vi "Helper Loop.vi"(8 "error in (no error)":errorcluster, 11 "RFSA DAQ in":refnum<class "RFSA DAQ.lvclass">) -> ()   [LabVIEW 2025, in "RFSA DAQ.lvlib" / "RFSA DAQ.lvclass"]
uses:
  RFSA DAQ.lvclass
  Helper Loop State.ctl
  <vilib>/Natan Biesmans/G2CPU GPU and CPU HPC Toolkit/G2CPU Libraries/Async IO/DMA Manager/DMA Manager.lvclass
  Configure VST.ctl
  <vilib>/Platform/TimedLoop/XDataNode/timing_clust.ctl
  <vilib>/Platform/TimedLoop/XDataNode/nitl_modes.ctl
  <vilib>/Platform/TimedLoop/XDataNode/wakeup.ctl
  RFSA DAQ.lvclass/RFSA DAQ.ctl
  <instrlib>/niRFSA/niRFSA.llb/niRFSA Acquisition Types.ctl
  Helper Loop Message.ctl
  Helper Loop Type.ctl
  TDMS DAQ/TDMS DAQ/Filled Buffers.ctl
  <vilib>/ActorFramework/Actor/Actor.lvclass/Actor.ctl
  <vilib>/ActorFramework/Message Enqueuer/Message Enqueuer.lvclass/Message Enqueuer.ctl
  DAQ Interface/DAQ Interface Messages/Process Filled Buffer Msg/Process Filled Buffer Msg.lvclass/Process Filled Buffer Msg.ctl
  780f3a39-6c74-4c42-b9e6-83f74691e199.vi
  780f3a39-6c74-4c42-b9e6-83f74691e199.vi/8445960e-929f-4715-bef2-3345fde3aa58.vi
  780f3a39-6c74-4c42-b9e6-83f74691e199.vi/206fbf6d-c74b-456c-96d5-ad8d28d1ffd8.vi
  780f3a39-6c74-4c42-b9e6-83f74691e199.vi/4cbfaf14-3946-45e6-aec4-337dfce7590f.vi
  780f3a39-6c74-4c42-b9e6-83f74691e199.vi/3076a2b9-925c-4d87-a949-889053232e05.vi
  <vilib>/ActorFramework/Message Enqueuer/Init from Existing Queue.vi
  <vilib>/ActorFramework/Message Enqueuer/Enqueue.vi
  <vilib>/Natan Biesmans/G2CPU GPU and CPU HPC Toolkit/G2CPU Libraries/Arrays/1DArray/s16/1D Array s16.lvclass
  DAQ Interface/DAQ Interface Messages/Process Filled Buffer Msg/Process Filled Buffer Msg.lvclass
  <instrlib>/niRFSA/niRFSA.llb/niRFSA Fetch IQ (1D I16 Data Ref).vi
  <vilib>/Natan Biesmans/G2CPU GPU and CPU HPC Toolkit/G2CPU Libraries/Runtime Licensing/G2CPU License Check.vi
  <vilib>/Natan Biesmans/G2CPU GPU and CPU HPC Toolkit/G2CPU Libraries/Manage Environment/G2CPU Get Backend.vi
  <vilib>/Utility/error.llb/Error Cluster From Error Code.vi
  <vilib>/Natan Biesmans/G2CPU GPU and CPU HPC Toolkit/G2CPU Libraries/Manage Environment/Find AF DLL.vi
  <vilib>/Natan Biesmans/G2CPU GPU and CPU HPC Toolkit/ArrayFire Driver/VIs/Run as Multi Device.vi
  <vilib>/Natan Biesmans/G2CPU GPU and CPU HPC Toolkit/G2CPU Libraries/Arrays/Array/G2CPU Set Array Pointer.vi
  <resource>/Natan Biesmans/G2CPU GPU and CPU HPC Toolkit/Garbage Collector/G2CPU DMAGarbageCollectorFGV.vi
  <vilib>/ActorFramework/Message Priority Queue/Priority Enqueue.vi
  <vilib>/platform/TimedLoop/XDataNode/XDataNode.xnode
  <vilib>/Natan Biesmans/G2CPU GPU and CPU HPC Toolkit/G2CPU Libraries/Arrays/Array/Array Prototype.lvclass
  <vilib>/ActorFramework/Message Enqueuer/Message Enqueuer.lvclass
  <vilib>/Platform/TimedLoop/XDataNode/XDNodeRunTimeDep.lvlib
  DAQ Interface/DAQ Interface/DAQ Interface.lvclass
  <vilib>/ActorFramework/Actor/Actor.lvclass
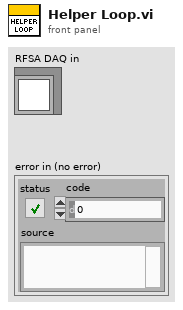
[diagram p1: front panel]
types:
  T1 = typedef "RFSA DAQ.lvlib/RFSA DAQ.lvclass/Helper Loop State.ctl" = cluster{"VST Config":T2, "DMA Manager":refnum<class "DMA Manager.lvclass">, "VST Handle":refnum<k15>, "Stop":bool}
  T2 = typedef "RFSA DAQ.lvlib/RFSA DAQ.lvclass/Configure VST.ctl" = cluster{"Samples to Read per Block":i32, "IQ rate (S/s)":dbl, "Carrier Frequency (Hz)":dbl, "Reference Level (dBm)":dbl, "Resource Name":refnum<k15>, "Clock Source":refnum<k15>, "Host DMA Buffer Size":i64}
  T3 = typedef "RFSA DAQ.lvlib/RFSA DAQ.lvclass/Helper Loop Message.ctl" = cluster{"Type":T4, "Payload":variant}
  T4 = typedef "RFSA DAQ.lvlib/RFSA DAQ.lvclass/Helper Loop Type.ctl" = enum16{"Configure", "Start", "Do", "Stop", "Clean", "Close"}
  T5 = typedef "DAQ Interface.lvlib/DAQ Interface.lvclass/Filled Buffers.ctl" = cluster{"DMA Manager":refnum<class "DMA Manager.lvclass">, "DMA Memory":refnum<data-value>, "Gain":dbl, "dt":dbl, "f0":dbl}
  T6 = typedef "XDNodeRunTimeDep.lvlib/timing_clust.ctl" = cluster{"Expected End [f-1]":u64, "Actual End [f-1]":u64, "Finished Late? [f-1]":bool, "Expected End [i-1]":u64, "Actual End [i-1]":u64, "Finished Late? [i-1]":bool, "Expected Start [i]":u64, "Actual Start [i]":u64, "Expected Start [f]":u64, "Actual Start [f]":u64, "Source Name":string, "Structure Name":string, "Period":i64, "Deadline":i64, "Offset":i64, "Start":i64, "Priority":i32, "Timeout":i32, "Mode":T7, "Wakeup Reason":T8, "Error":errorcluster, "Source Type":string, "Secondary Source Type":string, "Global End Time":u64, "Global Start Time":u64, "Frame Duration":u64, "Iteration Duration":u64, "Assigned CPU":i32, "I/O Scan Engine Mode":u32}
  T7 = typedef "XDNodeRunTimeDep.lvlib/nitl_modes.ctl" = enum32{"No Change", "Process missed periods, maintain original phase", "Discard missed periods, maintain original phase", "Process missed periods, ignore original phase", "Discard missed periods, ignore original phase"}
  T8 = typedef "XDNodeRunTimeDep.lvlib/wakeup.ctl" = enum32{"Normal", "Aborted", "Asynchronous wakeup", "Timing source error", "Timed loop error", "Timeout"}
  T9 = typedef "niRFSA Acquisition Types.ctl" = i32
  T10 = typedef "niRFSA wfmInfo.ctl" = cluster{"absolute timestamp":dbl, "relative timestamp":dbl, "dt":dbl, "actual samples read":i64, "offset":dbl, "gain":dbl, "reserved1":dbl, "reserved2":dbl}
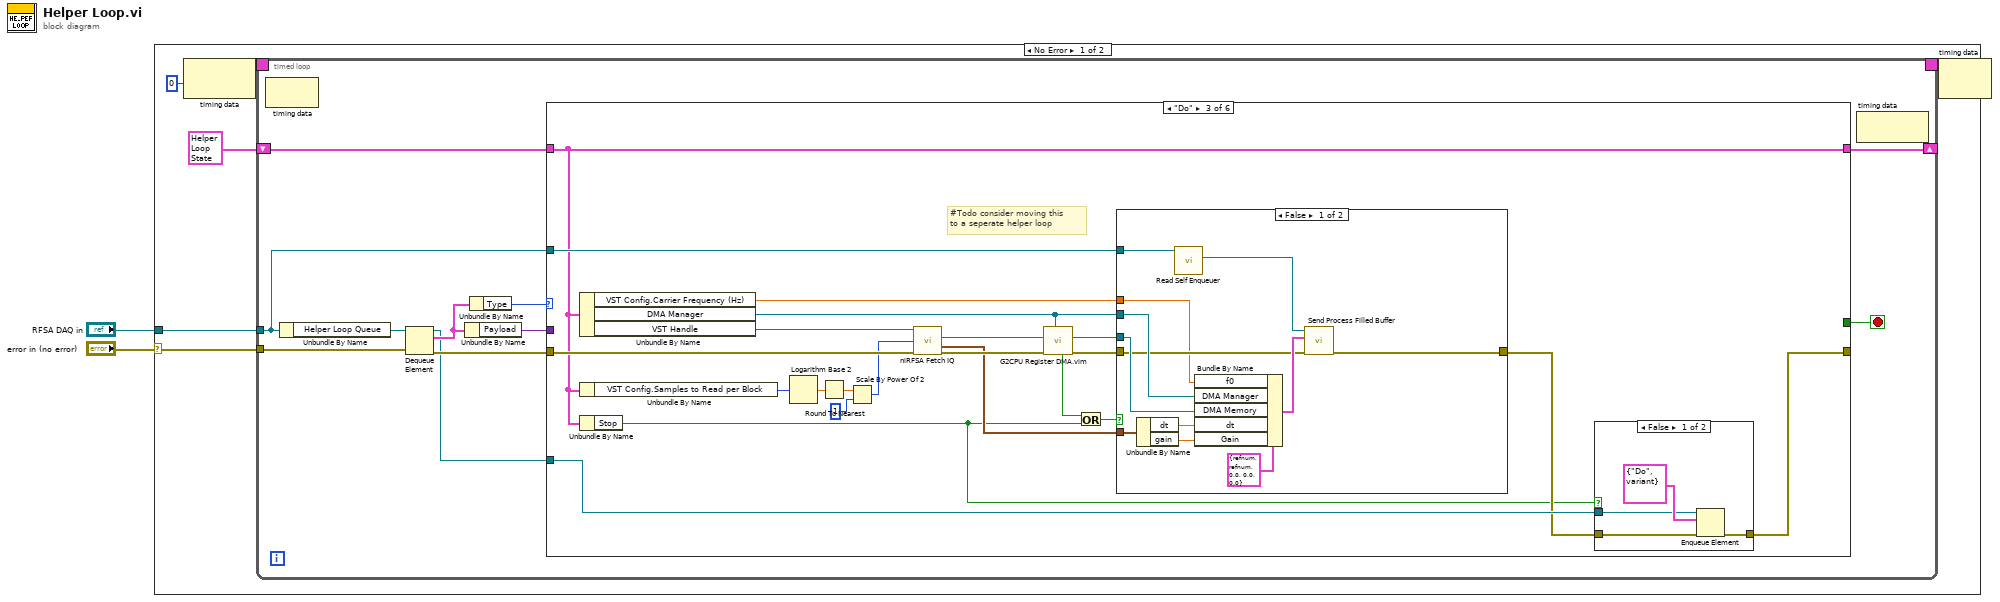
[diagram p0: block diagram]
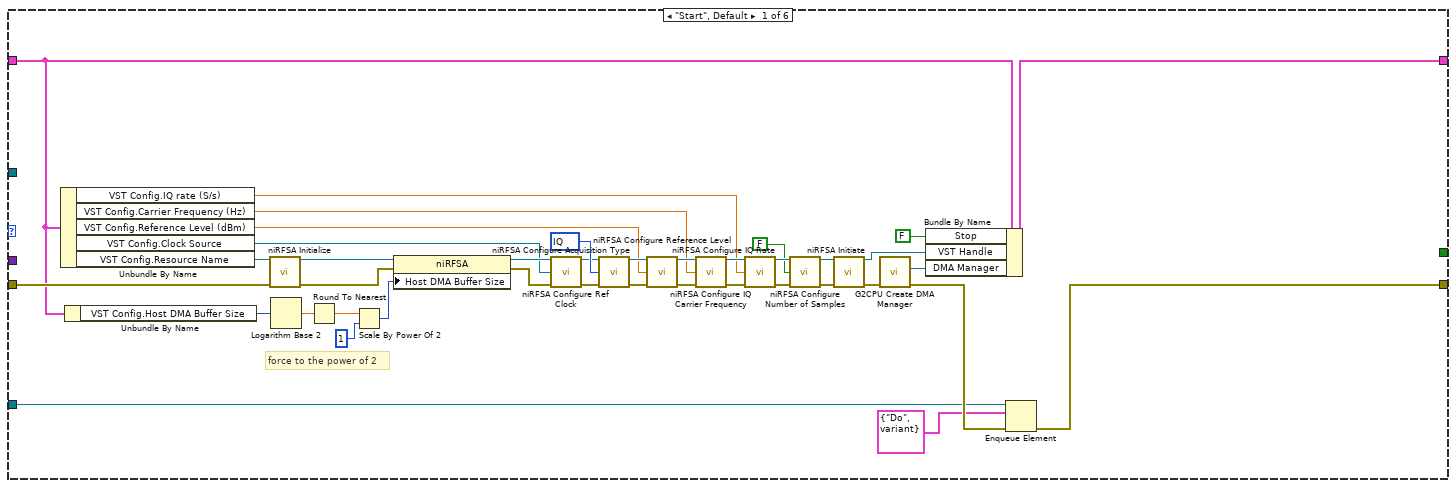
[diagram p2: hidden frame]
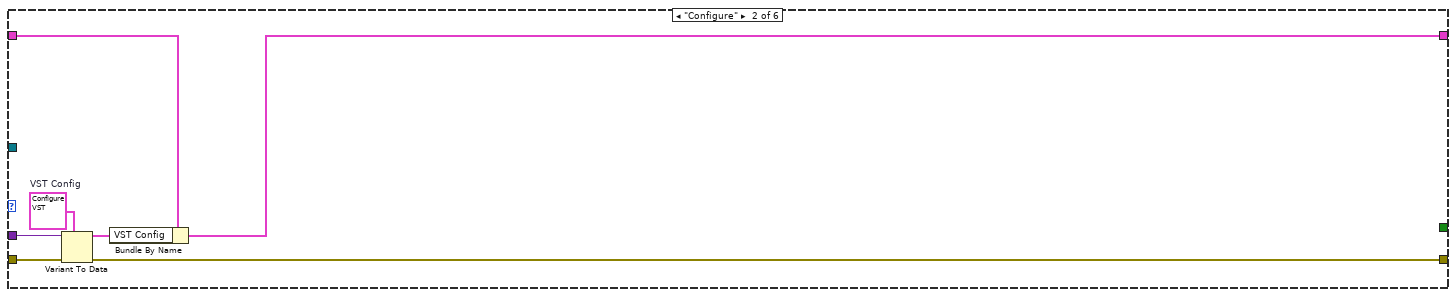
[diagram p3: hidden frame]
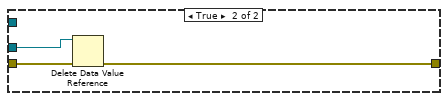
[diagram p5: hidden frame]
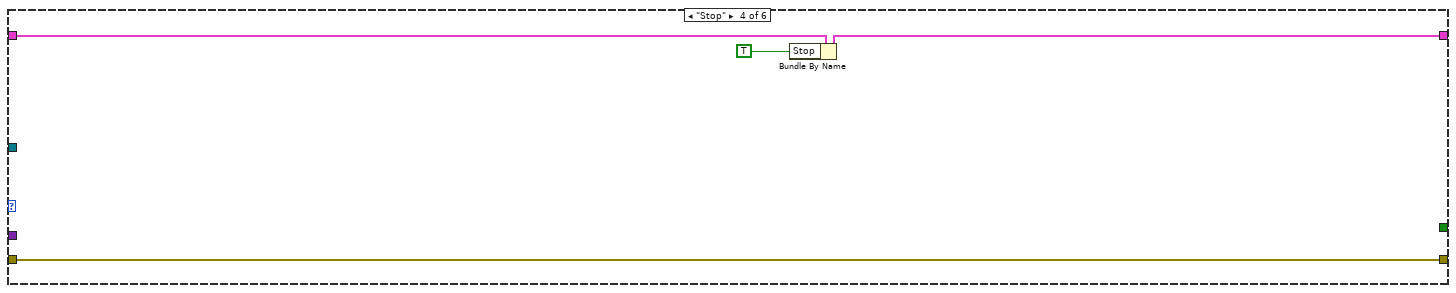
[diagram p6: hidden frame]
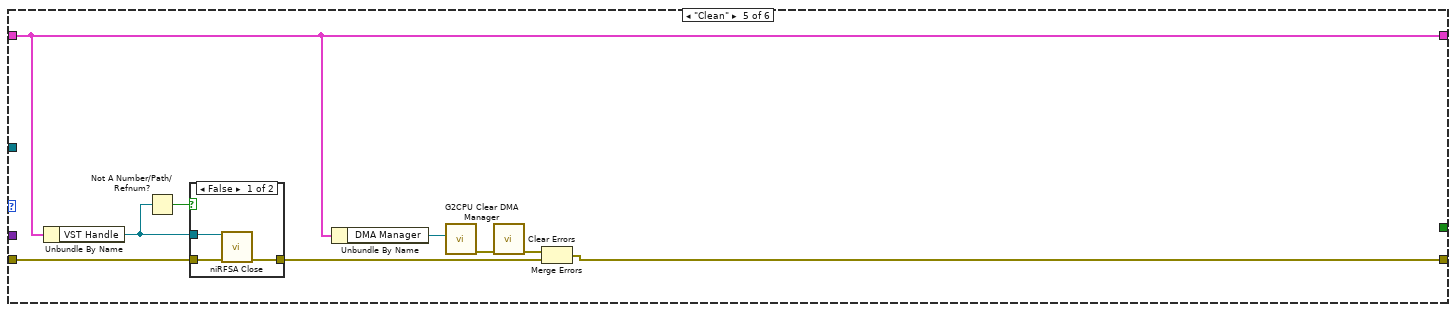
[diagram p7: hidden frame]
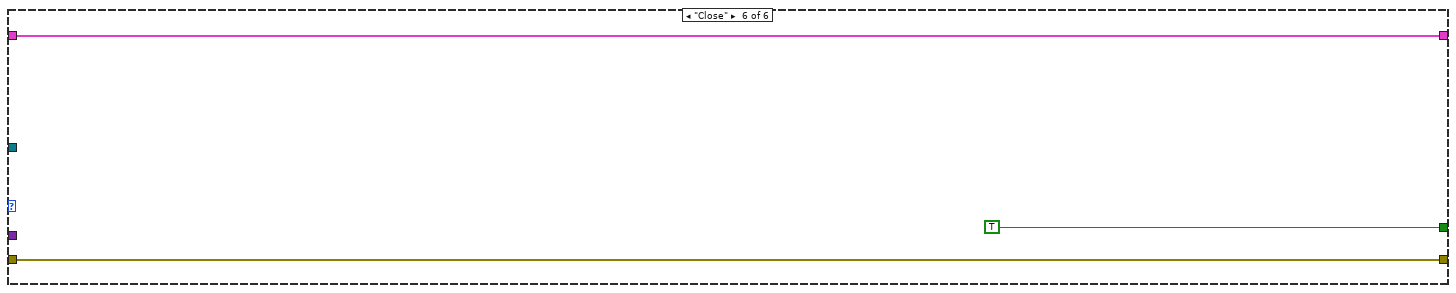
[diagram p9: hidden frame]
diagram:
  n1 = case shown="No Error" "error in (no error)" {
    selector: "error in (no error)" -> [w5 _]
    tunnel: "RFSA DAQ in" -> [w6 _]
    frame No Error {
      n2 = node-c288(i64 0 ("Period")) -> (w8:T6)
      n3 = timed-loop {
        timing: w8 -> [_]
        timing-out: [_] -> w7
        tunnel: w6 -> [w10]
        tunnel: w5 -> [w17]
        shift-right: [w12] -> _
        shift-left: T1 {"VST Config"={"Samples to Read per Block"=33554432, "IQ rate (S/s)"=1250000000.0, "Carrier Frequency (Hz)"=1000000000.0, "Reference Level (dBm)"=0.0, "Resource Name"="RFSA", "Clock Source"="OnboardClock", "Host DMA Buffer Size"=2000000000}, "DMA Manager"=refnum, "VST Handle"="", "Stop"=FALSE} ("State") -> [w11]
        stop <- w13 stop-if-true
        n4 = node-c288() -> ()  [unwired: 1 in, 1 out]
        n5 = Unbundle By Name(w10) -> ("Helper Loop Queue"=w19:refnum<queue>)
        n6 = Dequeue Element(queue=w19, error in (no error)=w17) -> (queue out=w9:refnum<queue>, element=w18:T3, error out=w15:errorcluster)  [unwired: 1 in, 1 out]
        n7 = Unbundle By Name(w18) -> ("Payload"=w14:variant)
        n8 = Unbundle By Name(w18) -> ("Type"=w16:T4)
        n9 = case shown="\"Do\"" w16 {
          tunnel: [w22 w62 w68 w110 w115 w127] -> _
          tunnel: w15 -> [w35 w63 w87 w110 w120 w127]
          tunnel: w14 -> [_ w64 _ _ _ _]
          tunnel: [_ _ _ _ _ TRUE] -> w13
          tunnel: [w27 w60 w71 w109 w116 w125] -> w12
          tunnel: w11 -> [w33 w61 w71 w111 w116 w125]
          tunnel: w10 -> [_ _ w74 _ _ _]
          tunnel: w9 -> [w21 _ w70 _ _ _]
          frame "Start", Default {
            w54 = T9 100 items=["IQ"=100, "Spectrum"=101] ("acquisition type")
            # "force to the power of 2"
            n10 = Unbundle By Name(w33) -> ("VST Config.IQ rate (S/s)"=w30:dbl, "VST Config.Carrier Frequency (Hz)"=w28:dbl, "VST Config.Reference Level (dBm)"=w29:dbl, "VST Config.Clock Source"=w31:refnum<k15>, "VST Config.Resource Name"=w34:refnum<k15>)
            n11 = Unbundle By Name(w33) -> ("VST Config.Host DMA Buffer Size"=w32:i64)
            n12 = call <instrlib>:"niRFSA Initialize.vi"("resource name"=w34, "error in"=w35) -> ("instrument handle out"=w45:refnum<k15>, "error out"=w38:errorcluster)  [unwired: 12 in]
            n13 = Logarithm Base 2(1:w32) -> (0:w39:dbl)
            n14 = Round To Nearest(number=w39) -> (nearest integer value=w40:dbl)
            n15 = Scale By Power Of 2(n=w40, x=u64 1) -> (x*2^n=w36:u64)
            n16 = property class="niRFSA"(reference=w45, error in=w38, "Host DMA Buffer Size"=w36) -> (reference out=w43:refnum<k15>, error out=w37:errorcluster)
            n17 = call <instrlib>:"niRFSA Configure Ref Clock.vi"("instrument handle"=w43, "clock source"=w31, "error in"=w37) -> ("instrument handle out"=w44:refnum<k15>, "error out"=w46:errorcluster)  [unwired: 11 in]
            n18 = call <instrlib>:"niRFSA Configure Acquisition Type.vi"("instrument handle"=w44, "acquisition type"=w54, "error in"=w46) -> ("instrument handle out"=w56:refnum<k15>, "error out"=w55:errorcluster)  [unwired: 11 in]
            n19 = call <instrlib>:"niRFSA Configure Reference Level.vi"("instrument handle"=w56, "reference level (dBm)"=w29, "error in"=w55) -> ("instrument handle out"=w57:refnum<k15>, "error out"=w58:errorcluster)  [unwired: 11 in]
            n20 = call <instrlib>:"niRFSA Configure IQ Carrier Frequency.vi"("instrument handle"=w57, "carrier frequency"=w28, "error in"=w58) -> ("instrument handle out"=w48:refnum<k15>, "error out"=w49:errorcluster)  [unwired: 11 in]
            n21 = call <instrlib>:"niRFSA Configure IQ Rate.vi"("instrument handle"=w48, "IQ rate (S/s)"=w30, "error in"=w49) -> ("instrument handle out"=w50:refnum<k15>, "error out"=w51:errorcluster)  [unwired: 11 in]
            n22 = call <instrlib>:"niRFSA Configure Number of Samples.vi"("instrument handle"=w50, "number of samples is finite"=FALSE, "error in"=w51) -> ("instrument handle out"=w53:refnum<k15>, "error out"=w52:errorcluster)  [unwired: 11 in]
            n23 = call <instrlib>:"niRFSA Initiate.vi"("instrument handle"=w53, "error in"=w52) -> ("instrument handle out"=w25:refnum<k15>, "error out"=w42:errorcluster)  [unwired: 12 in]
            n24 = call <vilib>:"G2CPU Create DMA Manager.vi"("error in (no error)"=w42) -> ("error out"=w23:errorcluster, "DMA Manager"=w26:refnum<class "DMA Manager.lvclass">)  [unwired: 9 in]
            n25 = Bundle By Name(cluster=w33, "Stop"=FALSE, "VST Handle"=w25, "DMA Manager"=w26) -> (w27:T1)
            n26 = Enqueue Element(queue=w21, element=T3 {"Type"=enum."Do", "Payload"=variant}, error in (no error)=w23) -> (error out=w22:errorcluster)  [unwired: 1 in, 2 out]
          }
          frame "Configure" {
            w65 = T2 {"Samples to Read per Block"=33554432, "IQ rate (S/s)"=1250000000.0, "Carrier Frequency (Hz)"=1000000000.0, "Reference Level (dBm)"=0.0, "Resource Name"="RFSA", "Clock Source"="OnboardClock", "Host DMA Buffer Size"=2000000000}  # VST Config
            n27 = Variant To Data(error in=w63, type=w65, Variant=w64) -> (data=w59:T2, error out=w62:errorcluster)
            n28 = Bundle By Name(cluster=w61, "VST Config"=w59) -> (w60:T1)
          }
          frame "Do" {
            # "#Todo consider moving this\nto a seperate helper loop"
            n29 = Unbundle By Name(w71) -> ("VST Config.Carrier Frequency (Hz)"=w66:dbl, "DMA Manager"=w73:refnum<class "DMA Manager.lvclass">, "VST Handle"=w84:refnum<k15>)
            n30 = Unbundle By Name(w71) -> ("VST Config.Samples to Read per Block"=w80:i32)
            n31 = Unbundle By Name(w71) -> ("Stop"=w67:bool)
            n32 = Logarithm Base 2(1:w80) -> (0:w81:dbl)
            n33 = Round To Nearest(number=w81) -> (nearest integer value=w82:dbl)
            n34 = Scale By Power Of 2(n=w82, x=u64 1) -> (x*2^n=w79:u64)
            n35 = call-poly <instrlib>:"niRFSA Fetch IQ.vi"("instrument handle"=w84, "samples to read (-1)"=w79, "error in"=w87) -> ("data value reference"=w85:refnum<data-value>, "wfm info"=w75:T10, "error out"=w86:errorcluster)  [unwired: 9 in, 1 out]
            n36 = call "G2CPU Register DMA.vim"("DMA Manager"=w73, "error in (no error)"=w86, "DMA Memory In"=w85) -> ("error out"=w77:errorcluster, "DMA Memory Out"=w76:refnum<data-value>, "Registered Memory Location"=w78:bool)  [unwired: 6 in]
            n37 = Or(x=w78, y=w67) -> (x .or. y?=w72:bool)
            n38 = case shown="False" w72 {
              tunnel: w77 -> [w97 w107]
              tunnel: w76 -> [w99 w106]
              tunnel: [w94 w105] -> w69
              tunnel: w75 -> [w104 _]
              tunnel: w74 -> [w96 _]
              tunnel: w73 -> [w100 _]
              tunnel: w66 -> [w93 _]
              frame False {
                n39 = Unbundle By Name(w104) -> ("dt"=w102:dbl, "gain"=w101:dbl)
                n40 = call <vilib>:"Read Self Enqueuer.vi"("Actor"=w96) -> ("Self Enqueuer"=w95:refnum<class "Message Enqueuer.lvclass">)  [unwired: 10 in]
                n41 = Bundle By Name(cluster=T5 {"DMA Manager"=refnum, "DMA Memory"=refnum, "Gain"=0.0, "dt"=0.0, "f0"=0.0} ("element"), "f0"=w93, "DMA Manager"=w100, "DMA Memory"=w99, "dt"=w102, "Gain"=w101) -> (w98:T5)
                n42 = call "Send Process Filled Buffer.vi"("error in (no error)"=w97, "Filled Buffers"=w98, "Message Enqueuer"=w95) -> ("error out"=w94:errorcluster)  [unwired: 7 in, 1 out]
              }
              frame True {
                n43 = Delete Data Value Reference(data value reference=w106, error in=w107) -> (error out=w105:errorcluster)  [unwired: 1 out]
              }
            }
            n44 = case shown="False" w67 {
              tunnel: w70 -> [w90 _]
              tunnel: w69 -> [w89 w92]
              tunnel: [w88 w92] -> w68
              frame False {
                n45 = Enqueue Element(queue=w90, element=T3 {"Type"=enum."Do", "Payload"=variant}, error in (no error)=w89) -> (error out=w88:errorcluster)  [unwired: 1 in, 2 out]
              }
              frame True {
              }
            }
          }
          frame "Stop" {
            n46 = Bundle By Name(cluster=w111, "Stop"=TRUE) -> (w109:T1)
          }
          frame "Clean" {
            n47 = Unbundle By Name(w116) -> ("VST Handle"=w118:refnum<k15>)
            n48 = Not A Number/Path/Refnum?(number/path/refnum=w118) -> (NaN/Path/Refnum?=w117:bool)
            n49 = case shown="False" w117 {
              tunnel: w120 -> [w123 w124]
              tunnel: [w122 w124] -> w119
              tunnel: w118 -> [w121 _]
              frame False {
                n50 = call <instrlib>:"niRFSA Close.vi"("instrument handle"=w121, "error in"=w123) -> ("error out"=w122:errorcluster)  [unwired: 13 in]
              }
              frame True {
              }
            }
            n51 = Unbundle By Name(w116) -> ("DMA Manager"=w112:refnum<class "DMA Manager.lvclass">)
            n52 = call <vilib>:"G2CPU Clear DMA Manager.vi"("DMA Manager"=w112) -> ("error out"=w113:errorcluster)  [unwired: 10 in]
            n53 = call <vilib>:"Clear Errors.vi"("error in (no error)"=w113) -> ("error out"=w114:errorcluster)  [unwired: 5 in, 1 out]
            n54 = Merge Errors(w114, w119) -> (w115:errorcluster)
          }
          frame "Close" {
          }
        }
        n55 = node-c288() -> ()  [unwired: 1 in, 1 out]
      }
      n56 = node-c288(w7) -> ()  [unwired: 1 out]
    }
    frame Error {
    }
  }
